vi "Read Element of TestSteps.vi"(8 "error in (no error)":errorcluster, 9 "UseCurrentTestPointer":bool, 10 "index":i32, 11 "TestSeqClass in":refnum<class "TestSeqClass.lvclass">) -> (0 "error out":errorcluster, 2 "TestMeasureStep.lvclass":refnum<class "TestMeasureStep.lvclass">, 3 "TestSeqClass out":refnum<class "TestSeqClass.lvclass">)   [LabVIEW 2019, in "TestSeqClass.lvclass"]
uses:
  TestSeqClass.lvclass
  TestMeasureStep/TestMeasureStep.lvclass
  TestSeqClass.lvclass/TestSeqClass.ctl
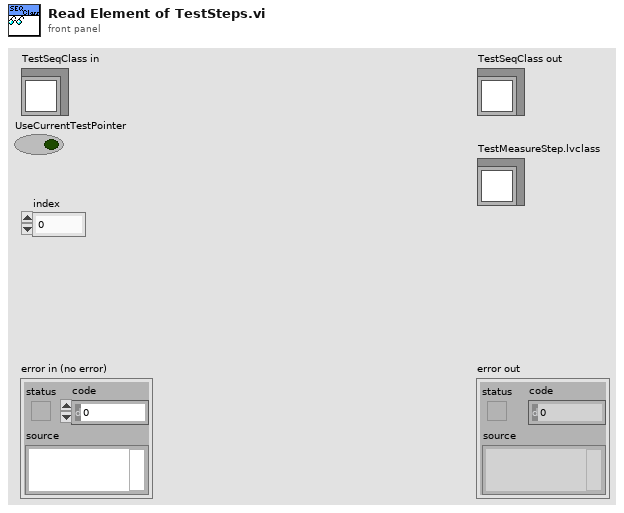
[diagram p1: front panel]
types:
  T1 = typedef "TestSeqType.ctl" = refnum<class "TestMeasureStep.lvclass">[]
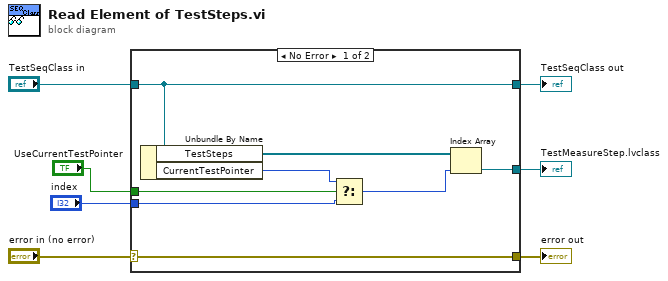
[diagram p0: block diagram]
diagram:
  n1 = case shown="No Error" "error in (no error)" {
    selector: "error in (no error)" -> [w15 w16]
    tunnel: [w15 w16] -> w6
    tunnel: [w14 w17] -> w4
    tunnel: "TestSeqClass in" -> [w14 w17]
    tunnel: [w12 _] -> w3
    tunnel: "index" -> [w11 _]
    tunnel: "UseCurrentTestPointer" -> [w8 _]
    frame No Error {
      n2 = Unbundle By Name(w14) -> ("TestSteps"=w13:T1, "CurrentTestPointer"=w9:i32)
      n3 = Select(t=w9, s=w8, f=w11) -> (s? t:f=w10:i32)
      n4 = Index Array(array=w13, index=w10) -> (element=w12:refnum<class "TestMeasureStep.lvclass">)
    }
    frame Error {
    }
  }
  "error out" <- w6
  "TestSeqClass out" <- w4
  "TestMeasureStep.lvclass" <- w3
